vi "DDE Open Conversation.vi"(8 "error in (no error)":errorcluster, 10 "topic":string, 11 "service":string) -> (0 "error out":errorcluster, 3 "conversation refnum":u32)   [LabVIEW 2018]
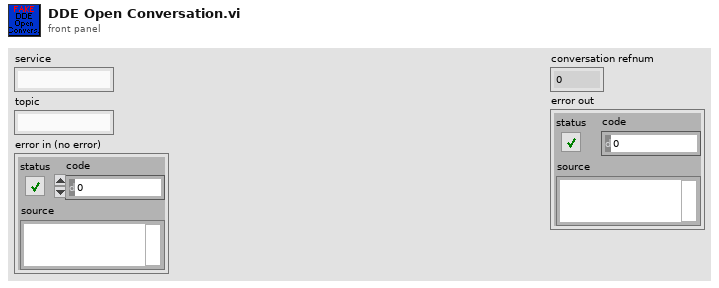
[diagram p1: front panel]
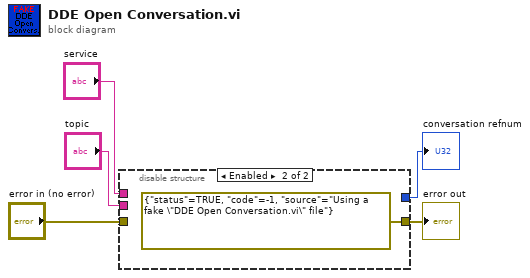
[diagram p0: block diagram]
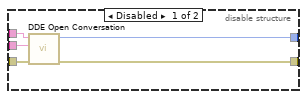
[diagram p2: hidden frame]
diagram:
  n1 = disable-structure shown="Enabled" {
    disable-tunnel: "service" -> [w10 _]
    disable-tunnel: "topic" -> [w9 _]
    disable-tunnel: "error in (no error)" -> [w8 _]
    disable-tunnel: [w7 _] -> w2
    disable-tunnel: [w6 errorcluster {"status"=TRUE, "code"=-1, "source"="Using a fake \"DDE Open Conversation.vi\" file"} ("error out")] -> w1
    frame Disabled {
      n2 = call "DDE Open Conversation.vi"("error in (no error)"=w8, "topic"=w9, "service"=w10) -> ("error out"=w6:errorcluster, "conversation refnum"=w7:u32)  [unwired: 5 in]
    }
    frame Enabled {
    }
  }
  "conversation refnum" <- w2
  "error out" <- w1
